vi "Write Data - Copy.vi"(0 "Bit In (SCLK & SYNC)":bool, 7 "Word In (DIN)":u32, 11 "error in (no error)":errorcluster, 12 "Socket Mask":u32, 13 "Line":T1) -> (15 "error out":errorcluster)   [LabVIEW 2017, in "FPGA-SRL.lvlib"]
uses:
  FPGA-SRL.lvlib
  <vilib>/eio/EIONode/EIONode.xnode
  Debug Global.vi
  <vilib>/rvi/eio/common/nirviEmuTemplateMethod_errors.vi
  Type Defs/Write Line Enum.ctl
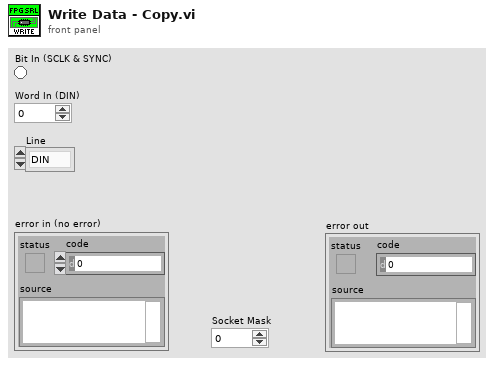
[diagram p1: front panel]
types:
  T1 = typedef "FPGA-SRL.lvlib/Write Line Enum.ctl" = enum16{"DIN", "SYNC", "SCLK"}
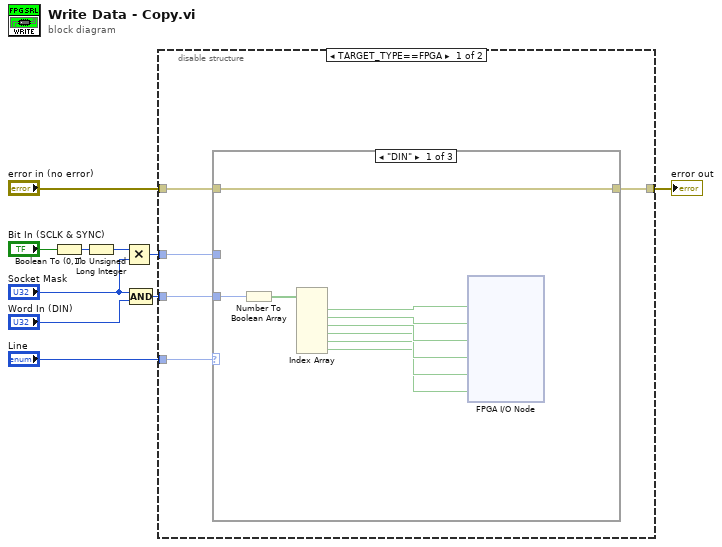
[diagram p0: block diagram]
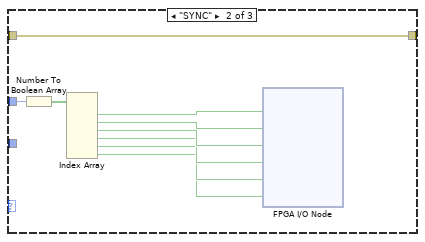
[diagram p2: hidden frame]
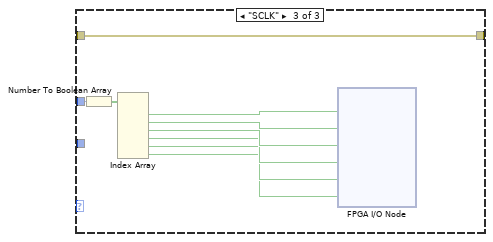
[diagram p3: hidden frame]
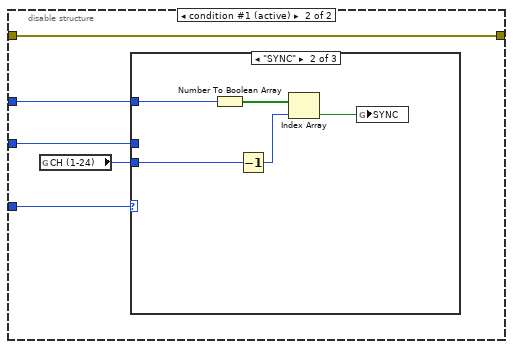
[diagram p4: hidden frame]
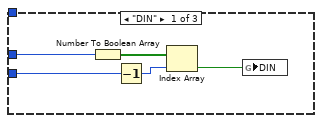
[diagram p5: hidden frame]
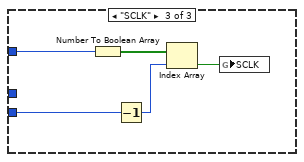
[diagram p6: hidden frame]
diagram:
  n1 = Boolean To (0,1)(Boolean="Bit In (SCLK & SYNC)") -> (0, 1=w4:i16)
  n2 = To Unsigned Long Integer(number=w4) -> (unsigned 32bit integer=w3:u32)
  n3 = Multiply(x=w3, y="Socket Mask") -> (x*y=w1:u32)
  n4 = Compound Arithmetic op=AND("Socket Mask", "Word In (DIN)") -> (w6:u32)
  n5 = disable-structure shown="TARGET_TYPE==FPGA" {
    disable-tunnel: "Line" -> [w15 w47]
    disable-tunnel: [w14 w46] -> w9
    disable-tunnel: "error in (no error)" -> [w13 w46]
    disable-tunnel: w6 -> [w12 w45]
    disable-tunnel: w1 -> [w11 w43]
    frame condition #0 {
      n6 = case shown="\"DIN\"" w15 {
        tunnel: [w24 w33 w40] -> w14
        tunnel: w13 -> [w24 w33 w40]
        tunnel: w12 -> [w22 _ _]
        tunnel: w11 -> [_ w32 w41]
        frame "DIN" {
          n7 = Number To Boolean Array(number=w22) -> (Boolean array=w23:bool[])
          n8 = Index Array(array=w23) -> (element #1=w21:bool, element #2=w20:bool, element #3=w19:bool, element #4=w18:bool, element #5=w17:bool, element #6=w16:bool)  [unwired: 6 in]
          n9 = xnode "FPGA I/O Node"("DIN_1"=w21, "DIN_2"=w20, "DIN_3"=w19, "DIN_4"=w18, "DIN_5"=w17, "DIN_6"=w16) -> ()  [unwired: 7 in, 7 out]
        }
        frame "SYNC" {
          n10 = Number To Boolean Array(number=w32) -> (Boolean array=w31:bool[])
          n11 = Index Array(array=w31) -> (element #1=w30:bool, element #2=w29:bool, element #3=w28:bool, element #4=w27:bool, element #5=w26:bool, element #6=w25:bool)  [unwired: 6 in]
          n12 = xnode "FPGA I/O Node"("SYNC_1"=w30, "SYNC_2"=w29, "SYNC_3"=w28, "SYNC_4"=w27, "SYNC_5"=w26, "SYNC_6"=w25) -> ()  [unwired: 6 in, 6 out]
        }
        frame "SCLK" {
          n13 = Number To Boolean Array(number=w41) -> (Boolean array=w42:bool[])
          n14 = Index Array(array=w42) -> (element #1=w39:bool, element #2=w38:bool, element #3=w37:bool, element #4=w36:bool, element #5=w35:bool, element #6=w34:bool)  [unwired: 6 in]
          n15 = xnode "FPGA I/O Node"("SCLK_1"=w39, "SCLK_2"=w38, "SCLK_3"=w37, "SCLK_4"=w36, "SCLK_5"=w35, "SCLK_6"=w34) -> ()  [unwired: 6 in, 6 out]
        }
      }
    }
    frame condition #1 (active) {
      n16 = global read "Debug Global.vi" "CH (1-24)"() -> (w44:i32)
      n17 = case shown="\"SYNC\"" w47 {
        tunnel: w45 -> [w49 _ _]
        tunnel: w44 -> [w48 w55 w60]
        tunnel: w43 -> [_ w53 w58]
        frame "DIN" {
          n18 = Number To Boolean Array(number=w49) -> (Boolean array=w52:bool[])
          n19 = Decrement(x=w48) -> (x-1=w50:i32)
          n20 = Index Array(array=w52, index=w50) -> (element=w51:bool)
          n21 = global write "Debug Global.vi" "DIN"(w51) -> ()
        }
        frame "SYNC" {
          n22 = Number To Boolean Array(number=w53) -> (Boolean array=w57:bool[])
          n23 = Decrement(x=w55) -> (x-1=w56:i32)
          n24 = Index Array(array=w57, index=w56) -> (element=w54:bool)
          n25 = global write "Debug Global.vi" "SYNC"(w54) -> ()
        }
        frame "SCLK" {
          n26 = Number To Boolean Array(number=w58) -> (Boolean array=w62:bool[])
          n27 = Decrement(x=w60) -> (x-1=w61:i32)
          n28 = Index Array(array=w62, index=w61) -> (element=w59:bool)
          n29 = global write "Debug Global.vi" "SCLK"(w59) -> ()
        }
      }
    }
  }
  "error out" <- w9
